vi "Get VI Checksums.vi"(8 "error in (no error)":errorcluster, 11 "NI_AB_API_Build in":refnum<class "NI_AB_API_Build.lvclass">) -> (0 "error out":errorcluster, 2 "VI Checksums":string[](array[string]), 3 "NI_AB_API_Build out":refnum<class "NI_AB_API_Build.lvclass">, 5 "Has errors?":bool=TRUE)   [LabVIEW 2020, in "NI_AB_API_Build.lvclass"]
uses:
  <vilib>/AppBuilder/AB_API/Build/NI_AB_API_Build.lvclass
  <vilib>/AppBuilder/AB_API/Build/NI_AB_API_Build.lvclass/NI_AB_API_Build.ctl
  <vilib>/AppBuilder/AB_Classes/Build/AB_Build.lvclass
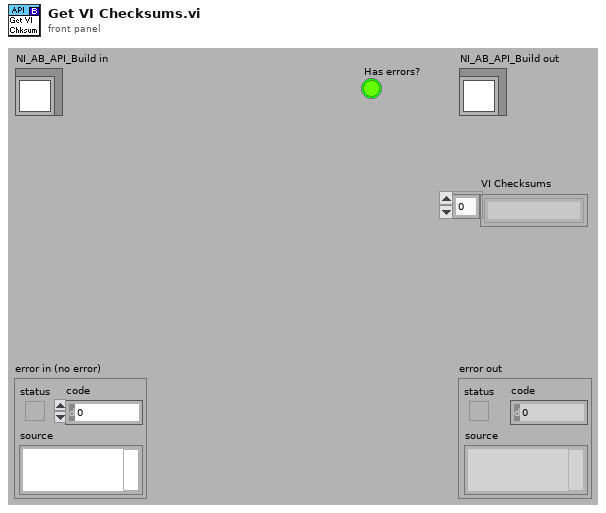
[diagram p1: front panel]
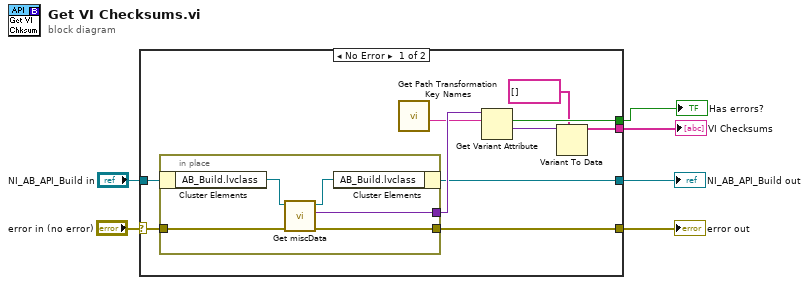
[diagram p0: block diagram]
diagram:
  n1 = case shown="No Error" "error in (no error)" {
    selector: "error in (no error)" -> [w16 w23]
    tunnel: [w15 w23] -> w5
    tunnel: [w11 w22] -> w3
    tunnel: "NI_AB_API_Build in" -> [w12 w22]
    tunnel: [w7 _] -> w1
    tunnel: [w14 _] -> w2
    frame No Error {
      n2 = in-place {
        in-place-border: w16 -> [w21]
        in-place-border: [w20] -> w15
        in-place-border: [w19] -> w13
        n3 = in-place-cluster #1(w12) -> ("AB_Build.lvclass"=w18:refnum<class "AB_Build.lvclass">)
        n4 = call-dynamic "Get miscData.vi"("error in (no error)"=w21, "AB_Build in"=w18) -> ("error out"=w20:errorcluster, "eng_miscData"=w19:variant, "AB_Build out"=w17:refnum<class "AB_Build.lvclass">)  [unwired: 7 in]
        n5 = in-place-cluster #1("AB_Build.lvclass"=w17) -> (w11:refnum<class "NI_AB_API_Build.lvclass">)
      }
      n6 = call <vilib>:"Get Path Transformation Key Names.vi"() -> ("VI Checksums"=w10:string)  [unwired: 9 in, 2 out]
      n7 = Get Variant Attribute(Variant=w13, name=w10) -> (found=w14:bool, value=w8:variant)  [unwired: 2 in, 2 out]
      n8 = Variant To Data(type=string[] [] ("VI Checksums"), Variant=w8) -> (data=w7:string[])  [unwired: 1 in, 1 out]
    }
    frame Error {
    }
  }
  "error out" <- w5
  "NI_AB_API_Build out" <- w3
  "VI Checksums" <- w1
  "Has errors?" <- w2
